vi "FITS_CloseFile.vi"(8 "error in":errorcluster, 11 "ref in":u64) -> (0 "error out":errorcluster, 2 "result":i32, 3 "ref out":u64)   [LabVIEW 2016]
uses:
  private/fitsLib/libfits_centos.so.4.0
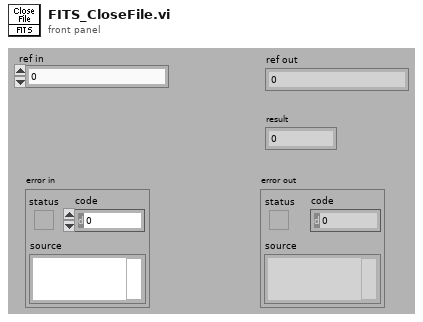
[diagram p1: front panel]
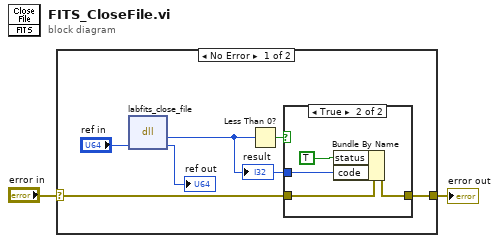
[diagram p0: block diagram]
diagram:
  n1 = case shown="No Error" "error in" {
    selector: "error in" -> [w7 w14]
    tunnel: [w6 w14] -> w1
    frame No Error {
      n2 = dll-call lib="home/harini/tcs/common_labview_cfitsio/private/fitsLib/libfits_centos.so.4.0" fn="labfits_close_file"("ref"="ref in") -> ("return type"=w5:i32, "ref"=→"ref out":u64)  [unwired: 3 in, 2 out]
      "result" <- w5
      n3 = Less Than 0?(x=w5) -> (x < 0?=w8:bool)
      n4 = case shown="True" w8 {
        tunnel: w7 -> [w9 w11]
        tunnel: [w9 w10] -> w6
        tunnel: w5 -> [_ w12]
        frame False {
        }
        frame True {
          n5 = Bundle By Name(cluster=w11, "status"=TRUE, "code"=w12) -> (w10:errorcluster)
        }
      }
    }
    frame Error {
    }
  }
  "error out" <- w1
